vi "Binary File Selection.vi"() -> (1 "cancelled":bool, 2 "klb paths":path[](array[path]), 3 "selected paths":path[](array[path]))   [LabVIEW 2013]
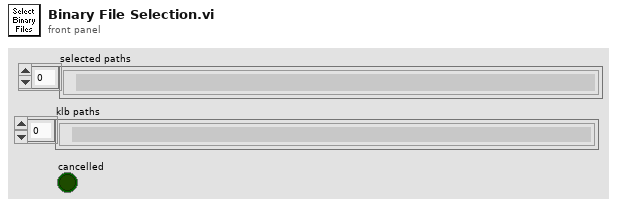
[diagram p1: front panel]
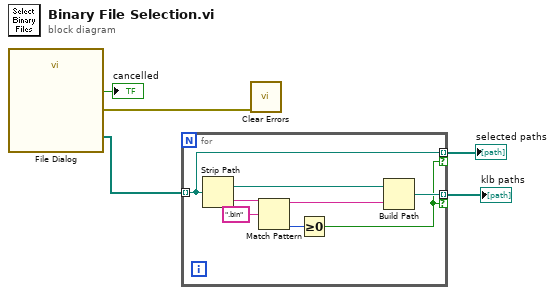
[diagram p0: block diagram]
diagram:
  n1 = call "File Dialog"() -> ("selected paths"=w5:path[], "cancelled"=→"cancelled":bool, "error out"=w2:errorcluster)  [unwired: 12 in, 1 out]
  n2 = for {
    tunnel: w5 -> [w8] mode=indexing
    tunnel: [w12] -> w1 mode=indexing if=w7
    tunnel: [w8] -> w3 mode=indexing if=w7
    n3 = Strip Path(path=w8) -> (stripped path=w13:path, name=w11:string)
    n4 = Match Pattern(string=w11, regular expression=".bin") -> (before substring=w6:string, offset past match=w9:i32)  [unwired: 1 in, 2 out]
    n5 = Greater Or Equal To 0?(x=w9) -> (x >= 0?=w7:bool)
    n6 = Build Path(base path=w13, name or relative path=w6) -> (appended path=w12:path)
  }
  "klb paths" <- w1
  "selected paths" <- w3
  n7 = call <vilib>:"Clear Errors.vi"("error in (no error)"=w2) -> ()  [unwired: 6 in, 1 out]
